vi "Remove Routing Channel State.vi"(8 "error in":errorcluster, 10 "state":string, 11 "routing channel in":T1 format="%.0x") -> (0 "error out":errorcluster, 3 "routing channel out":T1=18446744073709551615 format="%.0x")   [LabVIEW 2020, in "Routing and Faulting Scripting.lvlib"]
doc: "Removes the state with the specified name from the routing channel."
uses:
  Routing and Faulting Scripting.lvlib
  <vilib>/NI VeriStand/Custom Device API/Custom Device Item Ref.ctl
  <vilib>/Utility/error.llb/Error Cluster From Error Code.vi
  <vilib>/NI VeriStand/Custom Device API/Custom Device API.lvlib
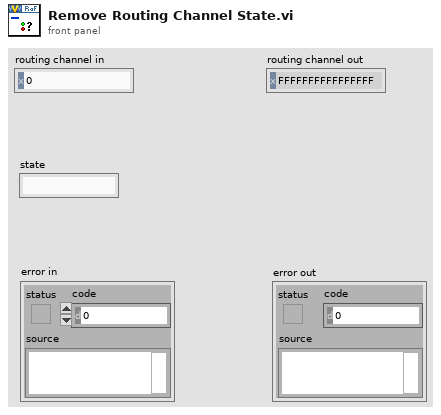
[diagram p1: front panel]
types:
  T1 = typedef "Custom Device API.lvlib/Custom Device Item Ref.ctl" = u64
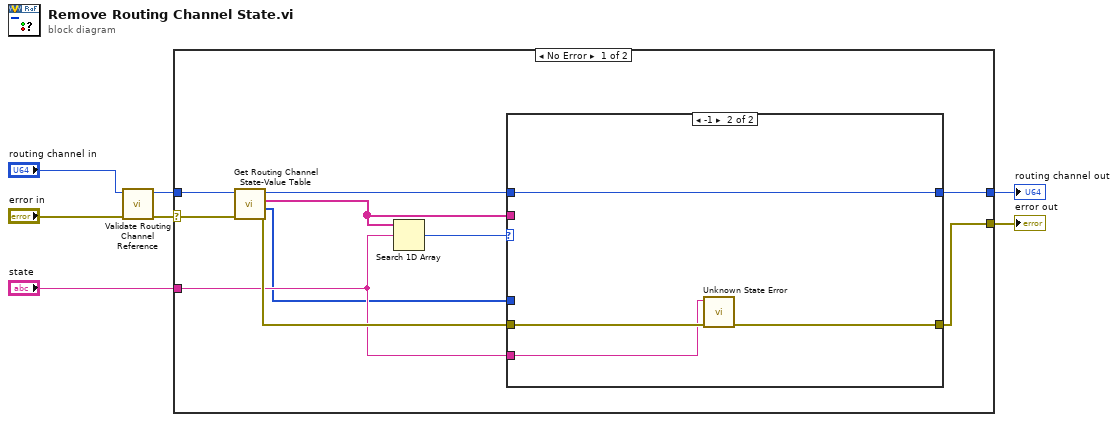
[diagram p0: block diagram]
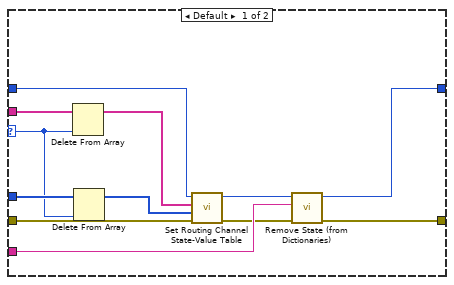
[diagram p2: hidden frame]
diagram:
  n1 = call "Validate Routing Channel Reference.vi"("error in"="error in", "routing channel in"="routing channel in") -> ("error out"=w3:errorcluster, "routing channel out"=w1:T1)  [unwired: 8 in]
  n2 = case shown="No Error" w3 {
    selector: w3 -> [w16 w35]
    tunnel: [w12 w35] -> w4
    tunnel: w1 -> [w17 w34]
    tunnel: [w13 w34] -> w6
    tunnel: "state" -> [w10 _]
    frame No Error {
      n3 = call "Get Routing Channel State-Value Table.vi"("error in"=w16, "routing channel in"=w17) -> ("error out"=w14:errorcluster, "state values"=w9:i32[], "state names"=w11:string[], "routing channel out"=w15:T1)  [unwired: 6 in]
      n4 = Search 1D Array(1D array=w11, element=w10) -> (index of element=w8:i32)  [unwired: 1 in]
      n5 = case shown="-1" w8 {
        selector: w8 -> [w20 _]
        tunnel: w15 -> [w29 w33]
        tunnel: w14 -> [w28 w32]
        tunnel: w9 -> [w21 _]
        tunnel: [w26 w33] -> w13
        tunnel: [w23 w31] -> w12
        tunnel: w11 -> [w22 _]
        tunnel: w10 -> [w25 w30]
        frame Default {
          # "State found, remove from table and Connections dictionary"
          n6 = Delete From Array(array=w22, index=w20) -> (array with subset deleted=w18:string[])  [unwired: 1 in, 1 out]
          n7 = Delete From Array(array=w21, index=w20) -> (array with subset deleted=w19:i32[])  [unwired: 1 in, 1 out]
          n8 = call "Set Routing Channel State-Value Table.vi"("error in"=w28, "state values"=w19, "state names"=w18, "routing channel in"=w29) -> ("error out"=w24:errorcluster, "routing channel out"=w27:T1)  [unwired: 6 in]
          n9 = call "Remove State (from Dictionaries).vi"("error in"=w24, "state"=w25, "routing channel in"=w27) -> ("error out"=w23:errorcluster, "routing channel out"=w26:T1)  [unwired: 7 in]
        }
        frame -1 {
          n10 = call "Unknown State Error.vi"("error in (no error)"=w32, "state"=w30) -> ("error out"=w31:errorcluster)  [unwired: 9 in]
        }
      }
    }
    frame Error {
    }
  }
  "routing channel out" <- w6
  "error out" <- w4
